vi "Configure Block Delimiter.vi"(8 "error in (no error)":errorcluster, 10 "Block Delimiter  (0: CRLF+EOI)":u16(ring) format="%.0g" items=["CRLF+EOI", "LF", "EOI"], 11 "VISA resource name":refnum<visa-resource-name>) -> (0 "error out":errorcluster, 3 "VISA resource name out":refnum<visa-resource-name>)   [LabVIEW 2017, in "ADCMT7451_ADC.lvlib"]
doc: "Configures the block delimiter on the instrument."
uses:
  ADCMT7451_ADC.lvlib
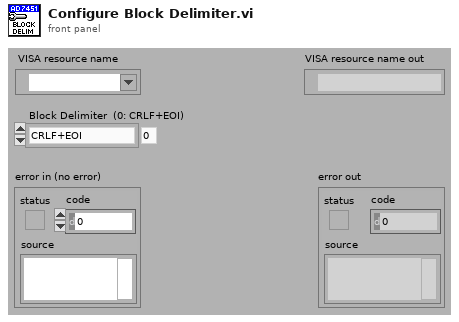
[diagram p1: front panel]
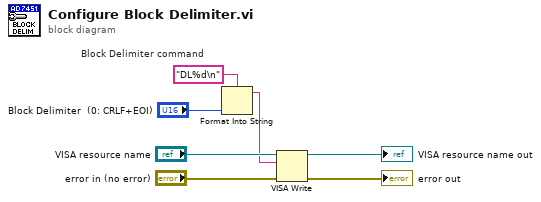
[diagram p0: block diagram]
diagram:
  w3 = "DL%d\n"  # Block Delimiter command
  n1 = Format Into String(format string=w3, "Block Delimiter  (0: CRLF+EOI)") -> (resulting string=w1:string)  [unwired: 2 in, 1 out]
  n2 = VISA Write(VISA resource name="VISA resource name", write buffer=w1, error in (no error)="error in (no error)") -> (VISA resource name out=→"VISA resource name out":refnum<visa-resource-name>, error out=→"error out":errorcluster)  [unwired: 1 out]
